vi "Copy 7zSD.SFX.vi"(8 "error in (no error)":errorcluster, 11 "PostBuildSupport in":refnum<class "PostBuildSupport.lvclass">) -> (0 "error out":errorcluster, 3 "PostBuildSupport out":refnum<class "PostBuildSupport.lvclass">)   [LabVIEW 2016, in "PostBuildSupport.lvclass"]
uses:
  PostBuildSupport.lvclass
  PostBuildSupport.lvclass/PostBuildSupport.ctl
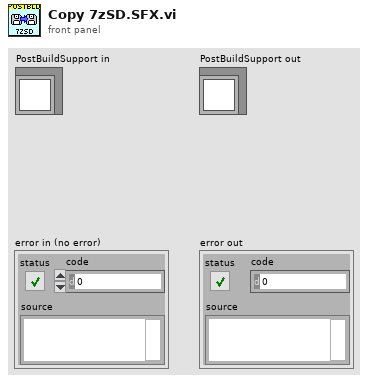
[diagram p1: front panel]
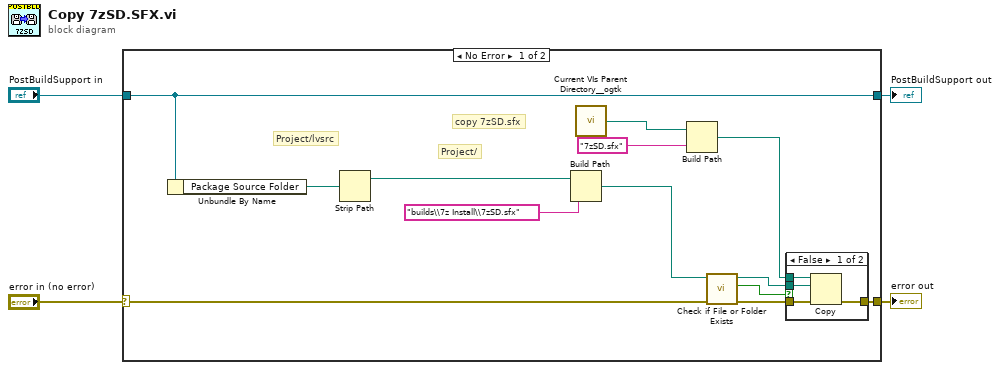
[diagram p0: block diagram]
diagram:
  n1 = case shown="No Error" "error in (no error)" {
    selector: "error in (no error)" -> [w8 w23]
    tunnel: [w15 w23] -> w4
    tunnel: "PostBuildSupport in" -> [w7 w24]
    tunnel: [w7 w24] -> w1
    frame No Error {
      # "Project/"
      # "Project/lvsrc"
      # "copy 7zSD.sfx"
      n2 = Unbundle By Name(w7) -> ("Package Source Folder"=w16:path)
      n3 = Strip Path(path=w16) -> (stripped path=w12:path)  [unwired: 1 out]
      n4 = Build Path(base path=w12, name or relative path="builds\\7z Install\\7zSD.sfx") -> (appended path=w6:path)
      n5 = call <userlib>:"Current VIs Parent Directory__ogtk.vi"() -> ("Parent Directory (+ Relative)"=w5:path)  [unwired: 5 in]
      n6 = Build Path(base path=w5, name or relative path="7zSD.sfx") -> (appended path=w13:path)
      n7 = call <vilib>:"Check if File or Folder Exists.vi"("error in (no error)"=w8, "path"=w6) -> ("error out"=w10:errorcluster, "file or folder exists?"=w9:bool, "dup path"=w11:path)  [unwired: 7 in]
      n8 = case shown="False" w9 {
        tunnel: [w21 w22] -> w15
        tunnel: w13 -> [w20 _]
        tunnel: w11 -> [w19 _]
        tunnel: w10 -> [w18 w22]
        frame False {
          n9 = Copy(8:w18, 10:w19, 11:w20) -> (0:w21:errorcluster)  [unwired: 2 in, 2 out]
        }
        frame True {
        }
      }
    }
    frame Error {
    }
  }
  "error out" <- w4
  "PostBuildSupport out" <- w1
